vi "qc5psm.vi"() -> ()   [LabVIEW 2020]
uses:
  <instrlib>/CAEN PSM/CAEN PSM.lvlib
panel:
  in  "Tab Control":enum32{"Page 1"}(tab)
  out "I monitor":dbl(graph)
  out "V monitor":dbl(graph)
  in  "VISA resource name":refnum<visa-resource-name>
  in  "Serial Configuration":T1={"Baud Rate"=115200, "Parity"=enum."None", "Data Bits"=8, "Stop Bits"=10, "Flow Control"=0} {"Flow Control" items=["None", "XON/XOFF", "RTS/CTS", "XON/XOFF & RTS/CTS", "DTR/DSR", "XON/XOFF & DTR/DSR"]; "Stop Bits" items=["1.0"=10, "1.5"=15, "2.0"=20]; "Data Bits" items=["7"=7, "8"=8]; "Baud Rate" items=["300"=300, "600"=600, "1200"=1200, "2400"=2400, "4800"=4800, "9600"=9600, "19200"=19200, "38400"=38400, "57600"=57600, "115200"=115200]}
  in  "Channel (0)":u8
  in  "Voltage ramp up (0 V/s)":u16 max=999
  in  "Voltage Max (0.0 V)":u16 max=9999
  in  "Req (Mohm)":dbl
  out "OVC":bool
  out "OVV":bool
  in  "stop":bool
  out "Channel Status Array":T2(array[cluster])
  out "Channel Status (decimal value)":i32[](array[numeric])
  out "Actual current level (Imon)":dbl
  out "Actual voltage level (Vmon)":dbl
  in  "Board Address":i8 max=31
  out "R calc":dbl
  in  "Vset":u16
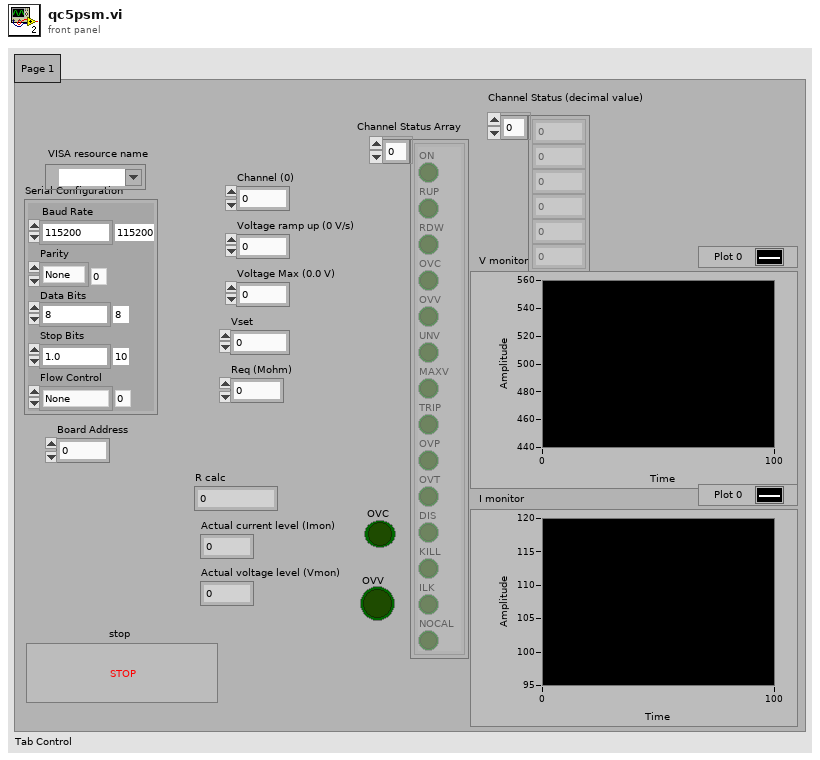
[diagram p1: front panel]
types:
  T1 = cluster{"Baud Rate":u32, "Parity":enum16{"None", "Odd", "Even", "Mark", "Space"}, "Data Bits":u16, "Stop Bits":u16, "Flow Control":u16}
  T2 = cluster{"ON":bool, "RUP":bool, "RDW":bool, "OVC":bool, "OVV":bool, "UNV":bool, "MAXV":bool, "TRIP":bool, "OVP":bool, "OVT":bool, "DIS":bool, "KILL":bool, "ILK":bool, "NOCAL":bool}[]
  T3 = typedef "CAEN PSM.lvlib/BoardHandle.ctl" = cluster{"VISA resource name":refnum<visa-resource-name>, "Board address":i8, "NChannels":u8}
  T4 = cluster{"ON":bool, "RUP":bool, "RDW":bool, "OVC":bool, "OVV":bool, "UNV":bool, "MAXV":bool, "TRIP":bool, "OVP":bool, "OVT":bool, "DIS":bool, "KILL":bool, "ILK":bool, "NOCAL":bool}
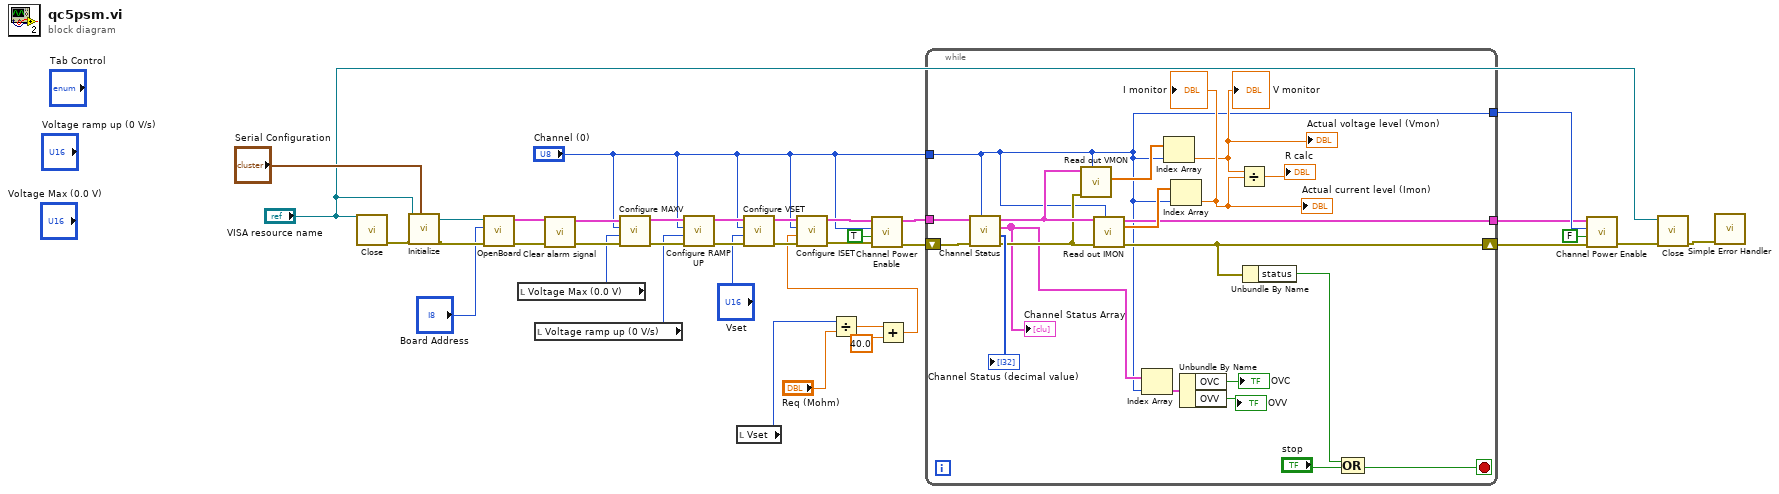
[diagram p0: block diagram]
diagram:
  n1 = call <instrlib>:"Close.vi"("VISA resource name"="VISA resource name") -> ("error out"=w6:errorcluster)  [unwired: 10 in]
  n2 = call <instrlib>:"Initialize.vi"("Serial Configuration"="Serial Configuration", "error in (no error)"=w6, "VISA resource name"="VISA resource name") -> ("error out"=w35:errorcluster, "VISA resource name out"=w34:refnum<visa-resource-name>)  [unwired: 7 in]
  n3 = call <instrlib>:"OpenBoard.vi"("error in (no error)"=w35, "Board Address"="Board Address", "VISA resource name"=w34) -> ("error out"=w32:errorcluster, "BoardHandle"=w33:T3)  [unwired: 7 in]
  n4 = local read "Voltage Max (0.0 V)"() -> (w27:u16)
  n5 = local read "Voltage ramp up (0 V/s)"() -> (w26:u16)
  n6 = call <instrlib>:"Clear alarm signal.vi"("error in (no error)"=w32, "BoardHandle"=w33) -> ("error out"=w30:errorcluster, "BoardHandle out"=w31:T3)  [unwired: 8 in]
  n7 = call <instrlib>:"Configure MAXV.vi"("error in (no error)"=w30, "Voltage Max (0.0 V)"=w27, "Channel (0)"="Channel (0)", "BoardHandle"=w31) -> ("error out"=w28:errorcluster, "BoardHandle out"=w29:T3)  [unwired: 6 in]
  n8 = call <instrlib>:"Configure RAMP UP.vi"("error in (no error)"=w28, "Voltage ramp up (0 V/s)"=w26, "Channel (0)"="Channel (0)", "BoardHandle"=w29) -> ("error out"=w25:errorcluster, "BoardHandle out"=w24:T3)  [unwired: 6 in]
  n9 = local read "Vset"() -> (w3:u16)
  n10 = call <instrlib>:"Configure VSET.vi"("error in (no error)"=w25, "Voltage Level (0.0 V)"="Vset", "Channel (0)"="Channel (0)", "BoardHandle"=w24) -> ("error out"=w23:errorcluster, "BoardHandle out"=w22:T3)  [unwired: 6 in]
  n11 = Divide(x=w3, y="Req (Mohm)") -> (x/y=w20:dbl)
  n12 = Add(x=w20, y=40.0) -> (x+y=w14:dbl)
  n13 = call <instrlib>:"Configure ISET.vi"("error in (no error)"=w23, "Current Limit (0.00 uA)"=w14, "Channel (0)"="Channel (0)", "BoardHandle"=w22) -> ("error out"=w18:errorcluster, "BoardHandle out"=w17:T3)  [unwired: 6 in]
  n14 = call <instrlib>:"Channel Power Enable.vi"("error in (no error)"=w18, "Enable (OFF)"=TRUE, "Channel (0)"="Channel (0)", "BoardHandle"=w17) -> ("error out"=w15:errorcluster, "BoardHandle out"=w16:T3)  [unwired: 6 in]
  n15 = while {
    tunnel: w16 -> [w56]
    shift-right: [w43] -> w13
    shift-left: w15 -> [w55]
    tunnel: "Channel (0)" -> [w37]
    tunnel: [w41] -> w11
    tunnel: [w37] -> w12
    stop <- w46 stop-if-true
    n16 = call <instrlib>:"Channel Status.vi"("Channel"=w37, "error in (no error)"=w55, "BoardHandle"=w56) -> ("error out"=w52:errorcluster, "Channel Status (decimal value)"=→"Channel Status (decimal value)":i32[], "Channel Status Array"=w50:T2, "BoardHandle out"=w53:T3)  [unwired: 5 in]
    "Channel Status Array" <- w50
    n17 = call <instrlib>:"Read out VMON.vi"("Channel"=w37, "error in (no error)"=w52, "BoardHandle"=w53) -> ("VMon values (V)"=w51:dbl[])  [unwired: 6 in, 2 out]
    n18 = call <instrlib>:"Read out IMON.vi"("Channel"=w37, "error in (no error)"=w52, "BoardHandle"=w53) -> ("error out"=w43:errorcluster, "IMon values (uA)"=w42:dbl[], "BoardHandle out"=w41:T3)  [unwired: 5 in, 1 out]
    n19 = Index Array(array=w50, index=w37) -> (element=w49:T4)
    n20 = Index Array(array=w51, index=w37) -> (element=w38:dbl)
    "Actual voltage level (Vmon)" <- w38
    "V monitor" <- w38
    n21 = Index Array(array=w42, index=w37) -> (element=w40:dbl)
    "Actual current level (Imon)" <- w40
    "I monitor" <- w40
    n22 = Unbundle By Name(w49) -> ("OVC"=→"OVC":bool, "OVV"=→"OVV":bool)
    n23 = Divide(x=w38, y=w40) -> (x/y=→"R calc":dbl)
    n24 = Unbundle By Name(w43) -> ("status"=w45:bool)
    n25 = Compound Arithmetic op=OR(w45, "stop") -> (w46:bool)
  }
  n26 = call <instrlib>:"Channel Power Enable.vi"("error in (no error)"=w13, "Enable (OFF)"=FALSE, "Channel (0)"=w12, "BoardHandle"=w11) -> ("error out"=w8:errorcluster)  [unwired: 6 in, 1 out]
  n27 = call <instrlib>:"Close.vi"("error in (no error)"=w8, "VISA resource name"="VISA resource name") -> ("error out"=w7:errorcluster)  [unwired: 9 in]
  n28 = call <vilib>:"Simple Error Handler.vi"("error in (no error)"=w7) -> ()  [unwired: 4 in, 5 out]
